vi "Constructor.vi"(8 "error in":errorcluster, 11 "Name":string) -> (0 "error out":errorcluster, 3 "CustomDataType":refnum<class "CustomData.lvclass">)   [LabVIEW 2021, in "ProligentXMLGenerator.lvlib" / "CustomData.lvclass"]
uses:
  CustomData.lvclass
  CustomData.lvclass/CustomData.ctl
  Data.ctl
  CustomElement/CustomElement.lvclass
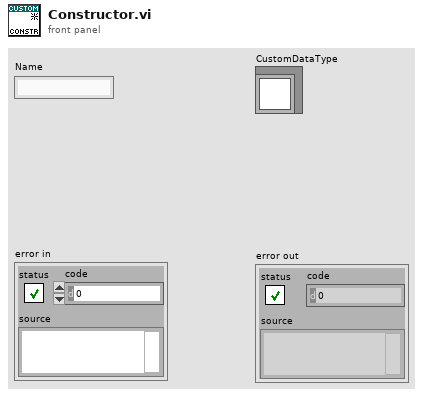
[diagram p1: front panel]
types:
  T1 = typedef "ProligentXMLGenerator.lvlib/CustomData.lvclass/Data.ctl" = cluster{"Name":string, "CustomElements":refnum<class "CustomElement.lvclass">[]}
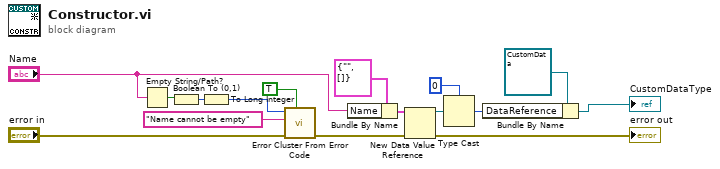
[diagram p0: block diagram]
diagram:
  n1 = Empty String/Path?(string/path="Name") -> (empty?=w7:bool)
  n2 = Boolean To (0,1)(Boolean=w7) -> (0, 1=w6:i16)
  n3 = To Long Integer(number=w6) -> (32bit integer=w5:i32)
  n4 = call <vilib>:"Error Cluster From Error Code.vi"("show call chain? (False)"=TRUE, "error in (no error)"="error in", "error message (\"\")"="Name cannot be empty" ("error message (\"\")"), "error code (0)"=w5) -> ("error out"=w2:errorcluster)  [unwired: 5 in]
  n5 = Bundle By Name(cluster=T1 {"Name"="", "CustomElements"=[]} ("Data"), "Name"="Name") -> (w12:T1)
  n6 = New Data Value Reference(data value=w12, error in=w2) -> (data value reference=w11:refnum<data-value>, error out=→"error out":errorcluster)
  n7 = Type Cast(type=u64 0, x=w11) -> (*(type *) &x=w9:u64)
  n8 = Bundle By Name(cluster=refnum<class "CustomData.lvclass"> refnum ("ProligentResultProcessor:CustomData"), "DataReference"=w9) -> (→"CustomDataType":refnum<class "CustomData.lvclass">)
